vi "HEWH Update Power Displays.vi"(8 "Error In":errorcluster, 11 "GEA Information In":T2 {"Water Heater GEA2 Data"."Hyperterminal Data"."CRC" format="%x"; "Water Heater GEA2 Data"."Hyperterminal Data"."Length" format="%x"; "Water Heater GEA2 Data"."Hyperterminal Data"."Command" format="%x"; "Water Heater GEA2 Data"."Hyperterminal Data"."Destination" format="%x"; "Water Heater GEA2 Data"."Hyperterminal Data"."Source" format="%x"; "Destination Address" format="%x"; "Source Address" format="%x"; "Command" format="%.0x"; "Data to send" format="%x"; "ReceivedData" format="%x"}) -> (0 "Error Out":errorcluster, 3 "POWER Out":T1)   [LabVIEW 2016]
uses:
  Washer HCC/Washer HCC NEWFI/Type Definitions/ViperHawk/ViperHawk Data.ctl
  Washer HCC/Washer HCC NEWFI/Type Definitions/ViperHawk/ViperHawk Diagnostic Data.ctl
  Utility/Save File/Public/Type Definitions/Save File Software Version.ctl
  Washer HCC/Washer HCC NEWFI/Type Definitions/ViperHawk/ViperHawk Search Control.ctl
  C:/Technology Lab/NI-2010/Trunk/Utility/LabVIEW GEA2 Toolkit v1.0.0.0/Appliance.NET/GeaCommunication.dll
  Utility/LabVIEW GEA2 Toolkit v1.0.0.0/Appliance.NET/GeaCommunication.dll
  Utility/LabVIEW GEA2 Toolkit v1.0.0.0/type defs/Data Out.ctl
  Utility/GEA2 Commands/HEWH/Type Definitions/GEA2 Commands WaterHeater GEA2 Data.ctl
  Utility/GEA2 Commands/HEWH/Type Definitions/GEA2 Commands Button Status.ctl
  Utility/GEA2 Commands/HEWH/Type Definitions/GEA2 Commands Status Query.ctl
  Utility/GEA2 Commands/HEWH/Type Definitions/GEA2 Commands Service Error Codes.ctl
  Type Definitions/HEWH Power Elements.ctl
  Utility/Save File/Save File.lvlib
  Utility/LabVIEW GEA2 Toolkit v1.0.0.0/library/GEA2_Toolkit.lvlib
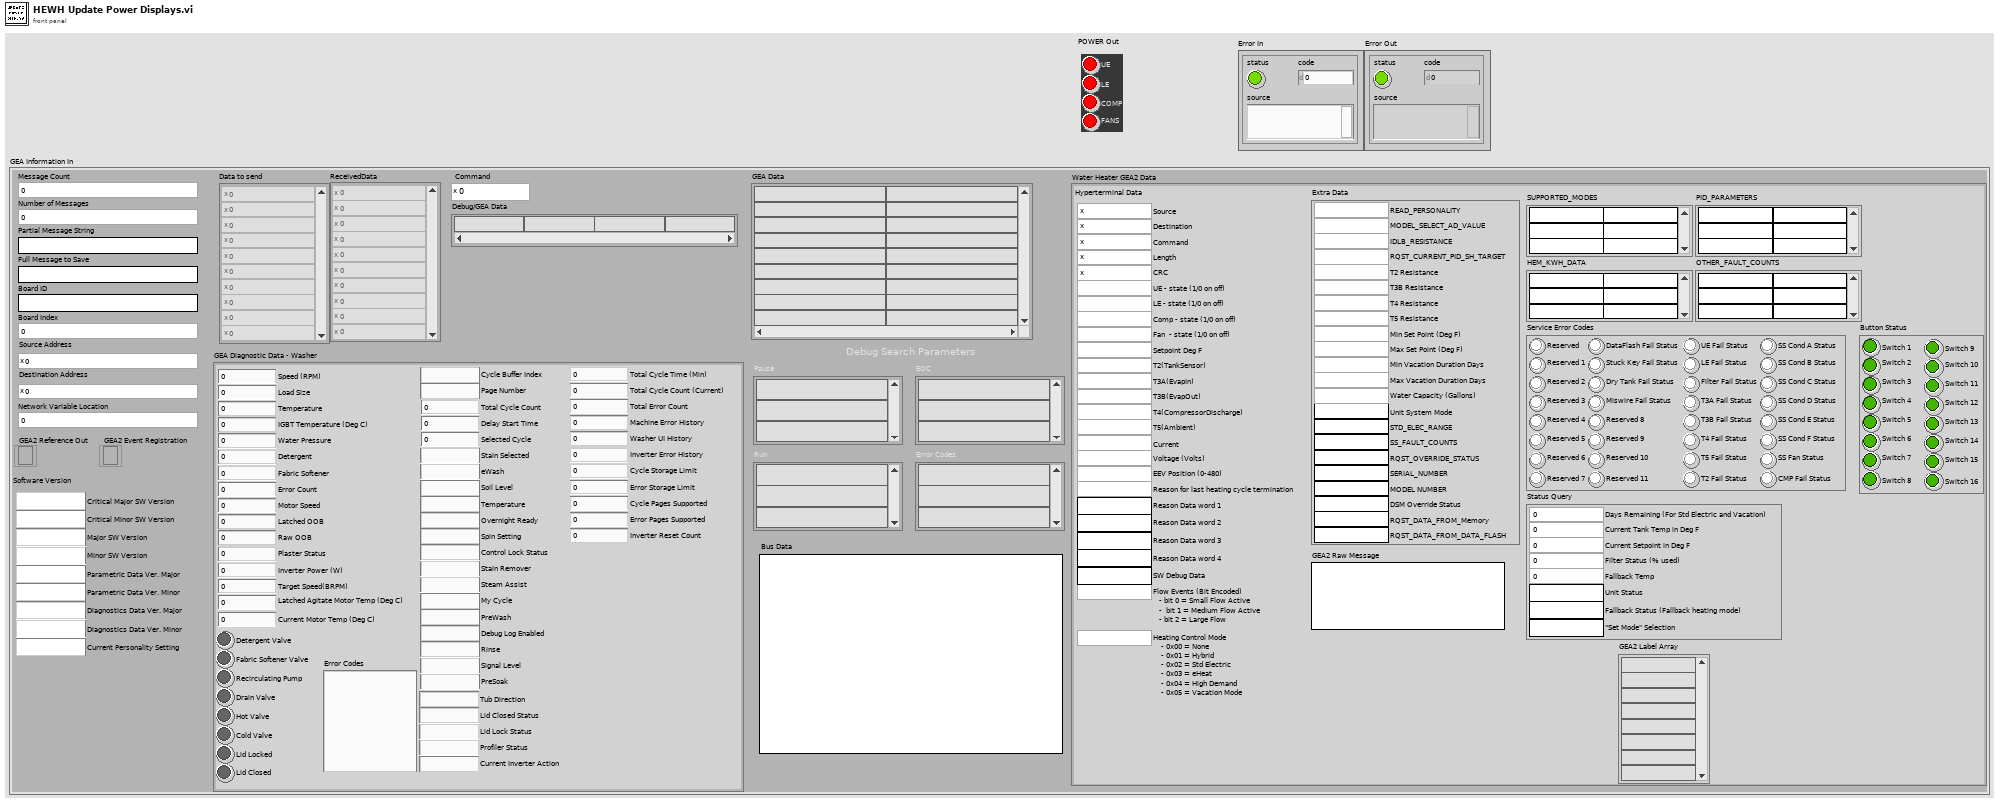
[diagram p1: front panel]
types:
  T1 = typedef "HEWH Power Elements.ctl" = cluster{"UE":bool, "LE":bool, "COMP":bool, "FANS":bool}
  T2 = typedef "ViperHawk Data.ctl" = cluster{"GEA Diagnostic Data - Washer":T3, "Software Version":T4, "Debug Search Parameters":T5, "Message Count":i32, "Number of Messages":i32, "Partial Message String":string, "Full Message to Save":string, "Board ID":string, "Board Index":i32, "Source Address":u8, "Destination Address":u8, "Data to send":u8[], "ReceivedData":u8[], "Debug/GEA Data":string[], "Command":u8, "GEA2 Reference Out":refnum<k24>, "GEA2 Event Registration":refnum<event-registration>, "Bus Data":string, "GEA Data":string[][], "Network Variable Location":i32, "Water Heater GEA2 Data":T6}
  T3 = typedef "ViperHawk Diagnostic Data.ctl" = cluster{"Speed (RPM)":u32, "Load Size":u32, "Temperature":u32, "Water Pressure":dbl, "Detergent":u32, "Fabric Softener":u32, "Tub Direction":string, "Detergent Valve":bool, "Fabric Softener Valve":bool, "Recirculating Pump":bool, "Drain Valve":bool, "Hot Valve":bool, "Cold Valve":bool, "Lid Closed Status":string, "Lid Lock Status":string, "Error Count":u32, "IGBT Temperature (Deg C)":u32, "Motor Speed":u32, "Latched OOB":u32, "Raw OOB":u32, "Plaster Status":u32, "Inverter Power (W)":u32, "Target Speed(BRPM)":u32, "Latched Agitate Motor Temp (Deg C)":u32, "Current Motor Temp (Deg C)":u32, "Profiler Status":string, "Current Inverter Action":string, "Error Codes":string, "Lid Locked":bool, "Lid Closed":bool, "9E Diagnostic Data":cluster{"Total Cycle Time (Min)":u32, "Total Cycle Count (Current)":u16, "Total Error Count":u16, "Machine Error History":u32, "Washer UI History":u32, "Inverter Error History":u32, "Cycle Storage Limit":u8, "Error Storage Limit":u8, "Cycle Pages Supported":u8, "Error Pages Supported":u8, "Inverter Reset Count":u16}, "9F Diagnostic Data":cluster{"Cycle Buffer Index":string, "Page Number":string, "Total Cycle Count":u32, "Delay Start Time":u32, "Stain Selected":string, "Selected Cycle":u32, "eWash":string, "Soil Level":string, "Temperature":string, "Overnight Ready":string, "Spin Setting":string, "Control Lock Status":string, "Stain Remover":string, "Steam Assist":string, "My Cycle":string, "PreWash":string, "Debug Log Enabled":string, "Rinse":string, "Signal Level":string, "PreSoak":string}}
  T4 = typedef "Save File.lvlib/Save File Software Version.ctl" = cluster{"Critical Major SW Version":string, "Critical Minor SW Version":string, "Major SW Version":string, "Minor SW Version":string, "Parametric Data Ver. Major":string, "Parametric Data Ver. Minor":string, "Diagnostics Data Ver. Major":string, "Diagnostics Data Ver. Minor":string, "Current Personality Setting":string}
  T5 = typedef "ViperHawk Search Control.ctl" = cluster{"Pause":string[], "Run":string[], "EOC":string[], "Error Codes":string[]}
  T6 = typedef "GEA2 Commands WaterHeater GEA2 Data.ctl" = cluster{"GEA2 Label Array":string[], "PID_PARAMETERS":string[][], "SUPPORTED_MODES":string[][], "Button Status":T7, "Status Query":T8, "Service Error Codes":T9, "HEM_KWH_DATA":string[][], "OTHER_FAULT_COUNTS":string[][], "GEA2 Raw Message":string, "Hyperterminal Data":cluster{"Source":u8, "Destination":u8, "Command":u8, "Length":u8, "CRC":u16, "UE - state (1/0 on off)":u8, "LE - state (1/0 on off)":u8, "Comp - state (1/0 on off)":u8, "Fan  - state (1/0 on off)":u8, "Setpoint Deg F":i32, "T2(TankSensor)":dbl, "T3A(EvapIn)":dbl, "T3B(EvapOut)":dbl, "T4(CompressorDischarge)":dbl, "T5(Ambient)":dbl, "Current":dbl, "Voltage (Volts)":u16, "EEV Position (0-480)":u16, "Reason for last heating cycle termination":u16, "Reason Data word 1":string, "Reason Data word 2":string, "Reason Data word 3":string, "Reason Data word 4":string, "SW Debug Data":string, "Flow Events (Bit Encoded)":u16, "Heating Control Mode":u16}, "Extra Data":cluster{"Water Capacity (Gallons)":u32, "Max Vacation Duration Days":u32, "Min Vacation Duration Days":u32, "Max Set Point (Deg F)":u32, "Min Set Point (Deg F)":u32, "T5 Resistance":u32, "T4 Resistance":u32, "T3B Resistance":u32, "T2 Resistance":u32, "STD_ELEC_RANGE":string, "SS_FAULT_COUNTS":string, "SERIAL_NUMBER":string, "READ_PERSONALITY":u8, "RQST_OVERRIDE_STATUS":string, "MODEL_SELECT_AD_VALUE":u32, "MODEL NUMBER":string, "IDLB_RESISTANCE":u32, "DSM Override Status":string, "RQST_DATA_FROM_Memory":string, "RQST_DATA_FROM_DATA_FLASH":string, "RQST_CURRENT_PID_SH_TARGET":u16, "Unit System Mode":string}}
  T7 = typedef "GEA2 Commands Button Status.ctl" = cluster{"Switch 1":bool, "Switch 2":bool, "Switch 3":bool, "Switch 4":bool, "Switch 5":bool, "Switch 6":bool, "Switch 7":bool, "Switch 8":bool, "Switch 9":bool, "Switch 10":bool, "Switch 11":bool, "Switch 12":bool, "Switch 13":bool, "Switch 14":bool, "Switch 15":bool, "Switch 16":bool}
  T8 = typedef "GEA2 Commands Status Query.ctl" = cluster{"Days Remaining (For Std Electric and Vacation)":u8, "Unit Status":string, "Current Tank Temp in Deg F":u8, "Current Setpoint in Deg F":u8, "Filter Status (% used)":u8, "Fallback Status (Fallback heating mode)":string, "Fallback Temp":u8, "\"Set Mode\" Selection":string}
  T9 = typedef "GEA2 Commands Service Error Codes.ctl" = cluster{"Reserved":bool, "Reserved 1":bool, "Reserved 2":bool, "Reserved 3":bool, "Reserved 4":bool, "Reserved 5":bool, "Reserved 6":bool, "Reserved 7":bool, "DataFlash Fail Status":bool, "Stuck Key Fail Status":bool, "Dry Tank Fail Status":bool, "Miswire Fail Status":bool, "Reserved 8":bool, "Reserved 9":bool, "Reserved 10":bool, "Reserved 11":bool, "UE Fail Status":bool, "LE Fail Status":bool, "Filter Fail Status":bool, "T3A Fail Status":bool, "T3B Fail Status":bool, "T4 Fail Status":bool, "T5 Fail Status":bool, "T2 Fail Status":bool, "SS Cond A Status":bool, "SS Cond B Status":bool, "SS Cond C Status":bool, "SS Cond D Status":bool, "SS Cond E Status":bool, "SS Cond F Status":bool, "SS Fan Status":bool, "CMP Fail Status":bool}
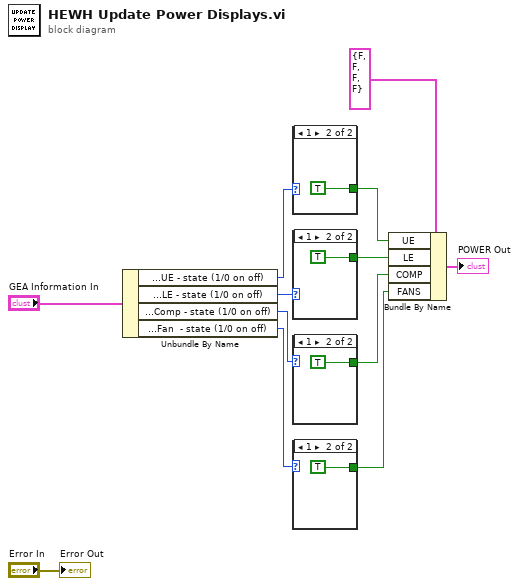
[diagram p0: block diagram]
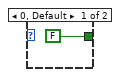
[diagram p2: hidden frame]
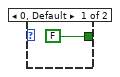
[diagram p3: hidden frame]
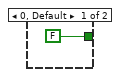
[diagram p4: hidden frame]
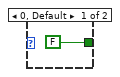
[diagram p5: hidden frame]
diagram:
  n1 = Unbundle By Name("GEA Information In") -> ("Water Heater GEA2 Data.Hyperterminal Data.UE - state (1/0 on off)"=w11:u8, "Water Heater GEA2 Data.Hyperterminal Data.LE - state (1/0 on off)"=w7:u8, "Water Heater GEA2 Data.Hyperterminal Data.Comp - state (1/0 on off)"=w6:u8, "Water Heater GEA2 Data.Hyperterminal Data.Fan  - state (1/0 on off)"=w5:u8)
  n2 = case shown="1" w11 {
    tunnel: [FALSE TRUE] -> w8
    frame 0, Default {
    }
    frame 1 {
    }
  }
  n3 = case shown="1" w7 {
    tunnel: [FALSE TRUE] -> w4
    frame 0, Default {
    }
    frame 1 {
    }
  }
  n4 = case shown="1" w6 {
    tunnel: [FALSE TRUE] -> w3
    frame 0, Default {
    }
    frame 1 {
    }
  }
  n5 = case shown="1" w5 {
    tunnel: [FALSE TRUE] -> w2
    frame 0, Default {
    }
    frame 1 {
    }
  }
  n6 = Bundle By Name(cluster=T1 {"UE"=FALSE, "LE"=FALSE, "COMP"=FALSE, "FANS"=FALSE} ("POWERA"), "UE"=w8, "LE"=w4, "COMP"=w3, "FANS"=w2) -> (→"POWER Out":T1)
  "Error Out" <- "Error In"
